vi "Simple UDP - Receiver_.vi"() -> ()   [LabVIEW 2020]
doc: "UDP协议与TCP的区别在于UDP不包括发送数据包信息的错误检查，因此无法保证接收端是否已接收所发数据。\n\nUDP可用于“广播”数据至整个网络，只需指定可包括全部的IP地址(255.255.255.255)以便发送信息至整个网络。 由于路由器或其他网络硬件通常拒绝转发超过一定点的数据，在实际应用中广播范围可能存在限制。"
panel:
  out "波形图表 6":waveform(i32)(graph)
  out "输出波形":waveform(i32)
  in  "停止 2":bool
  out "波形图表 5":i32[](graph)
  in  "服务器关闭":string="服务器VI关闭了连接。"
  # "概述：演示使用UDP函数通过UDP连接接收数据。\n操作步骤：\n1.确保已运行Simple UDP - Sender.vi。\n2.运行VI。\n3.单击停止按钮停止VI。"
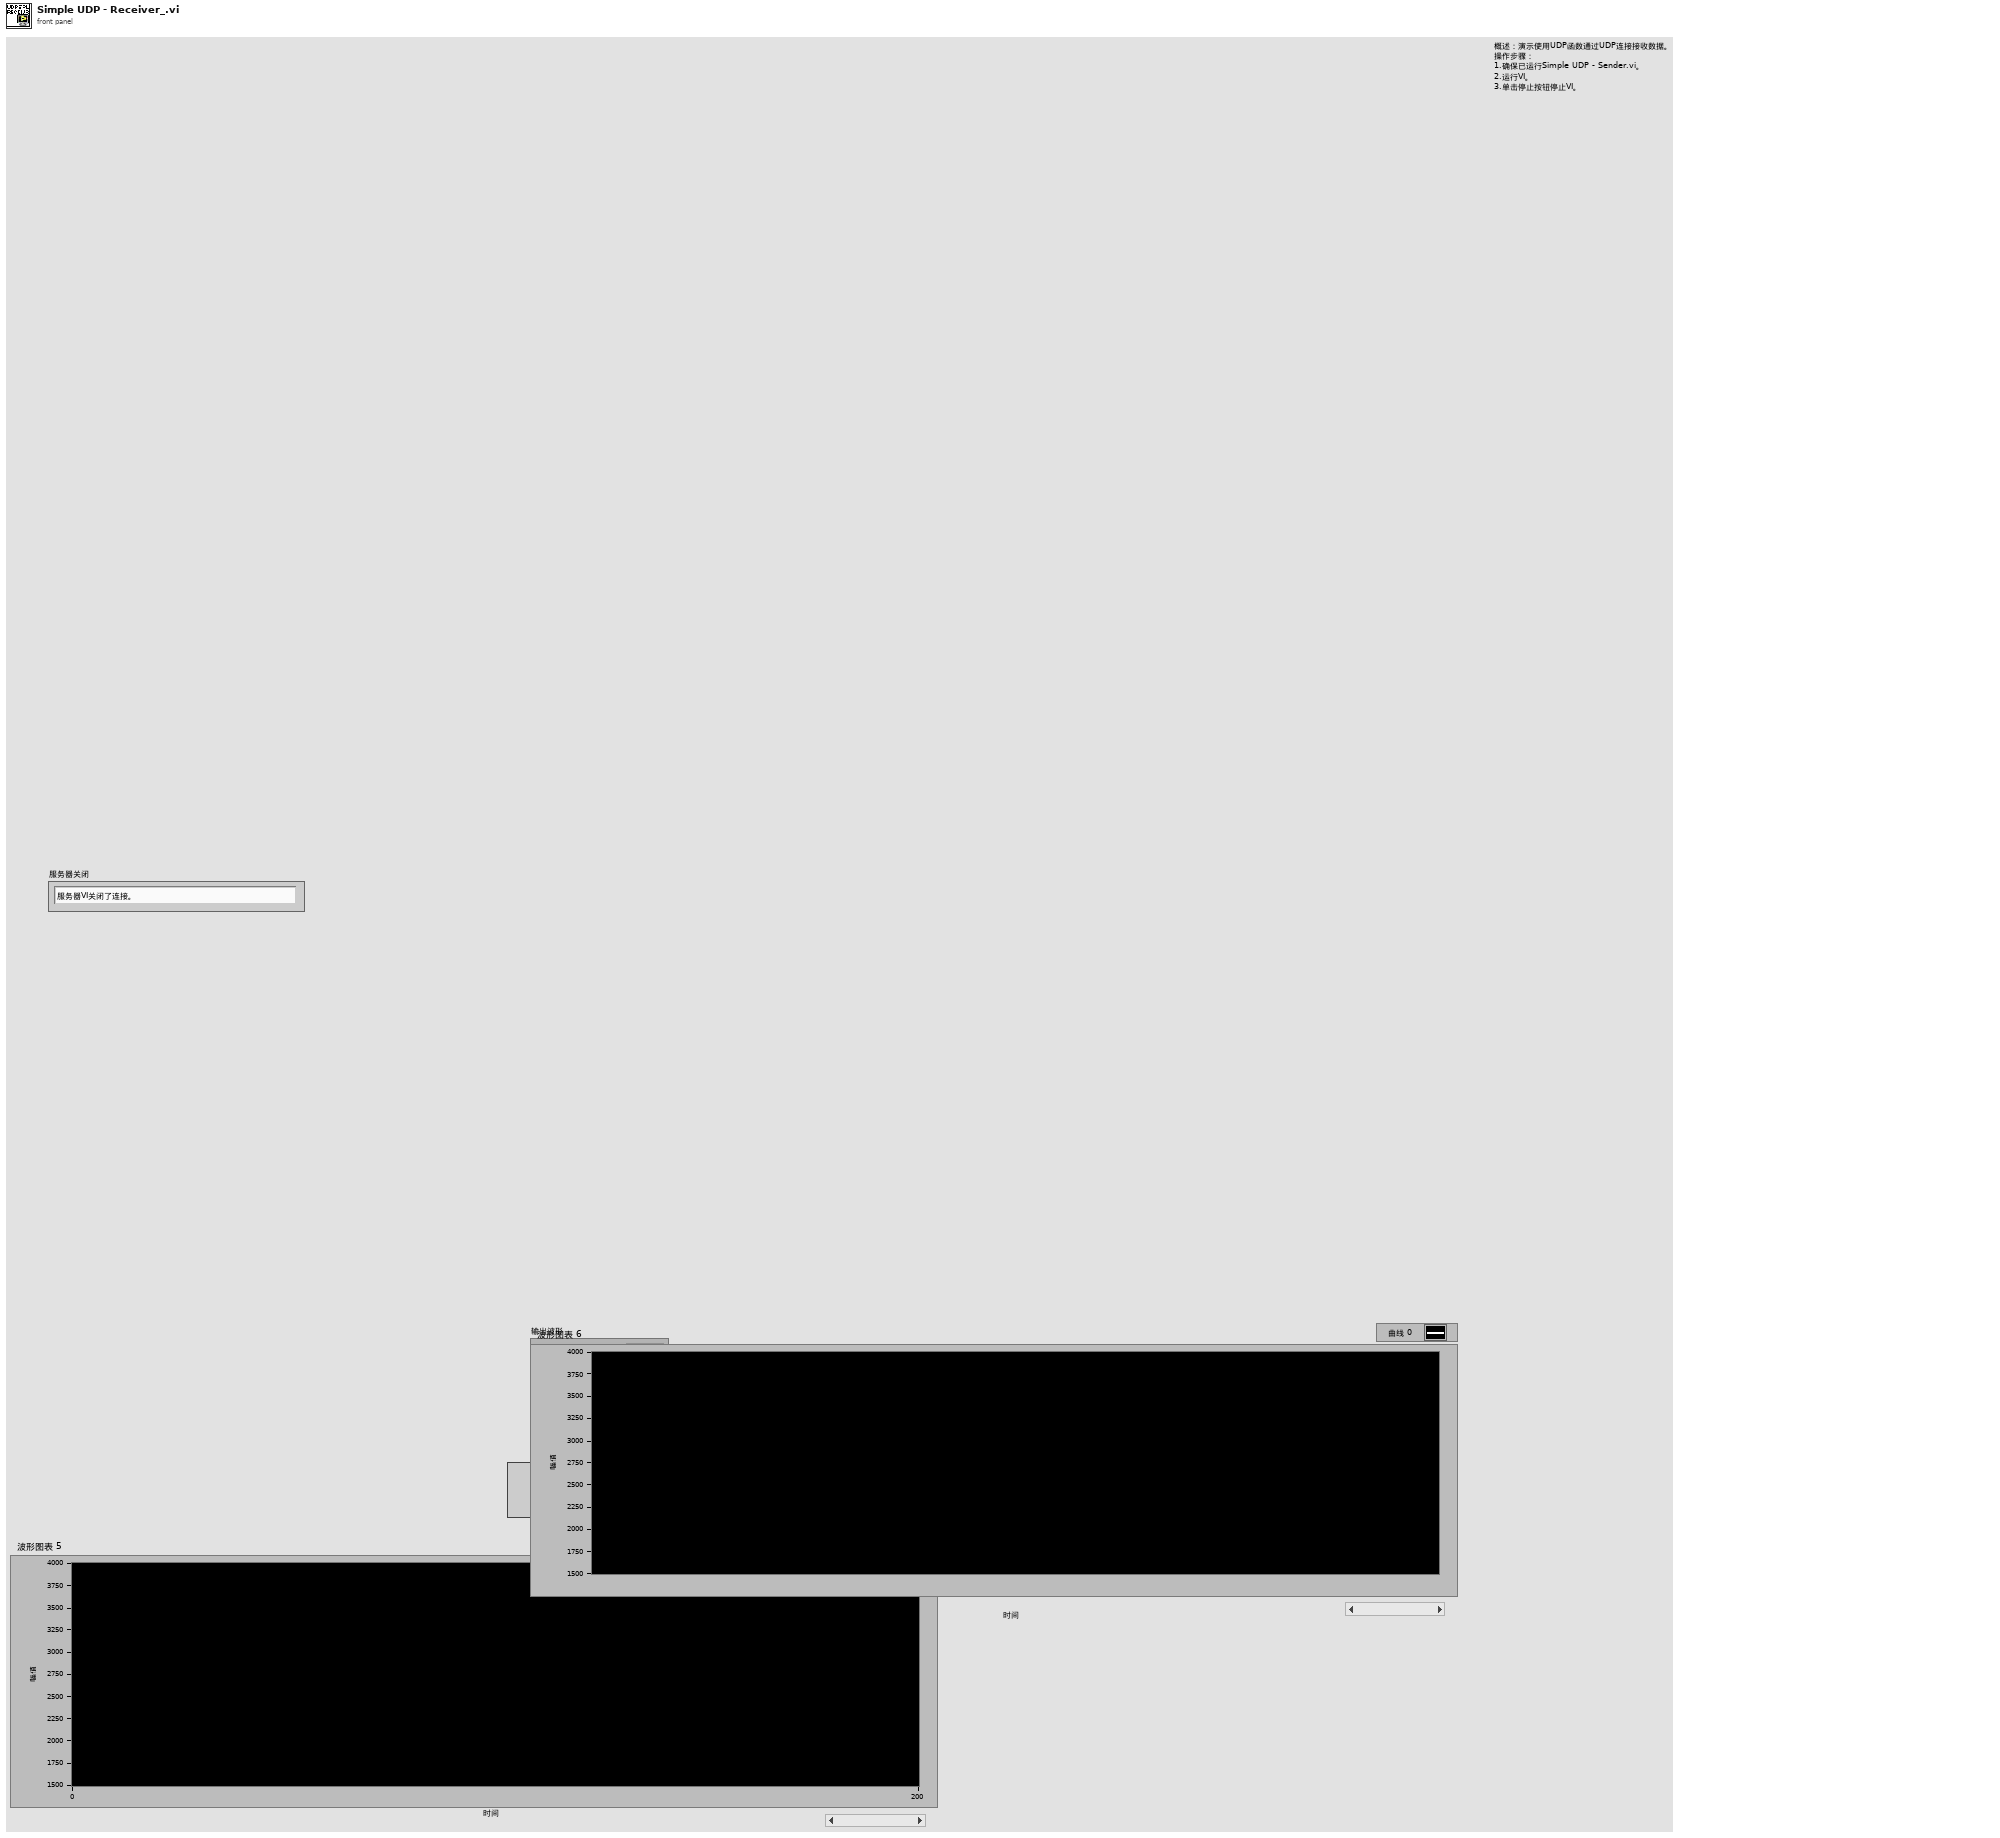
[diagram p1: front panel]
types:
  T1 = enum16{"open", "open or create", "create or replace", "create", "open (read-only)"}
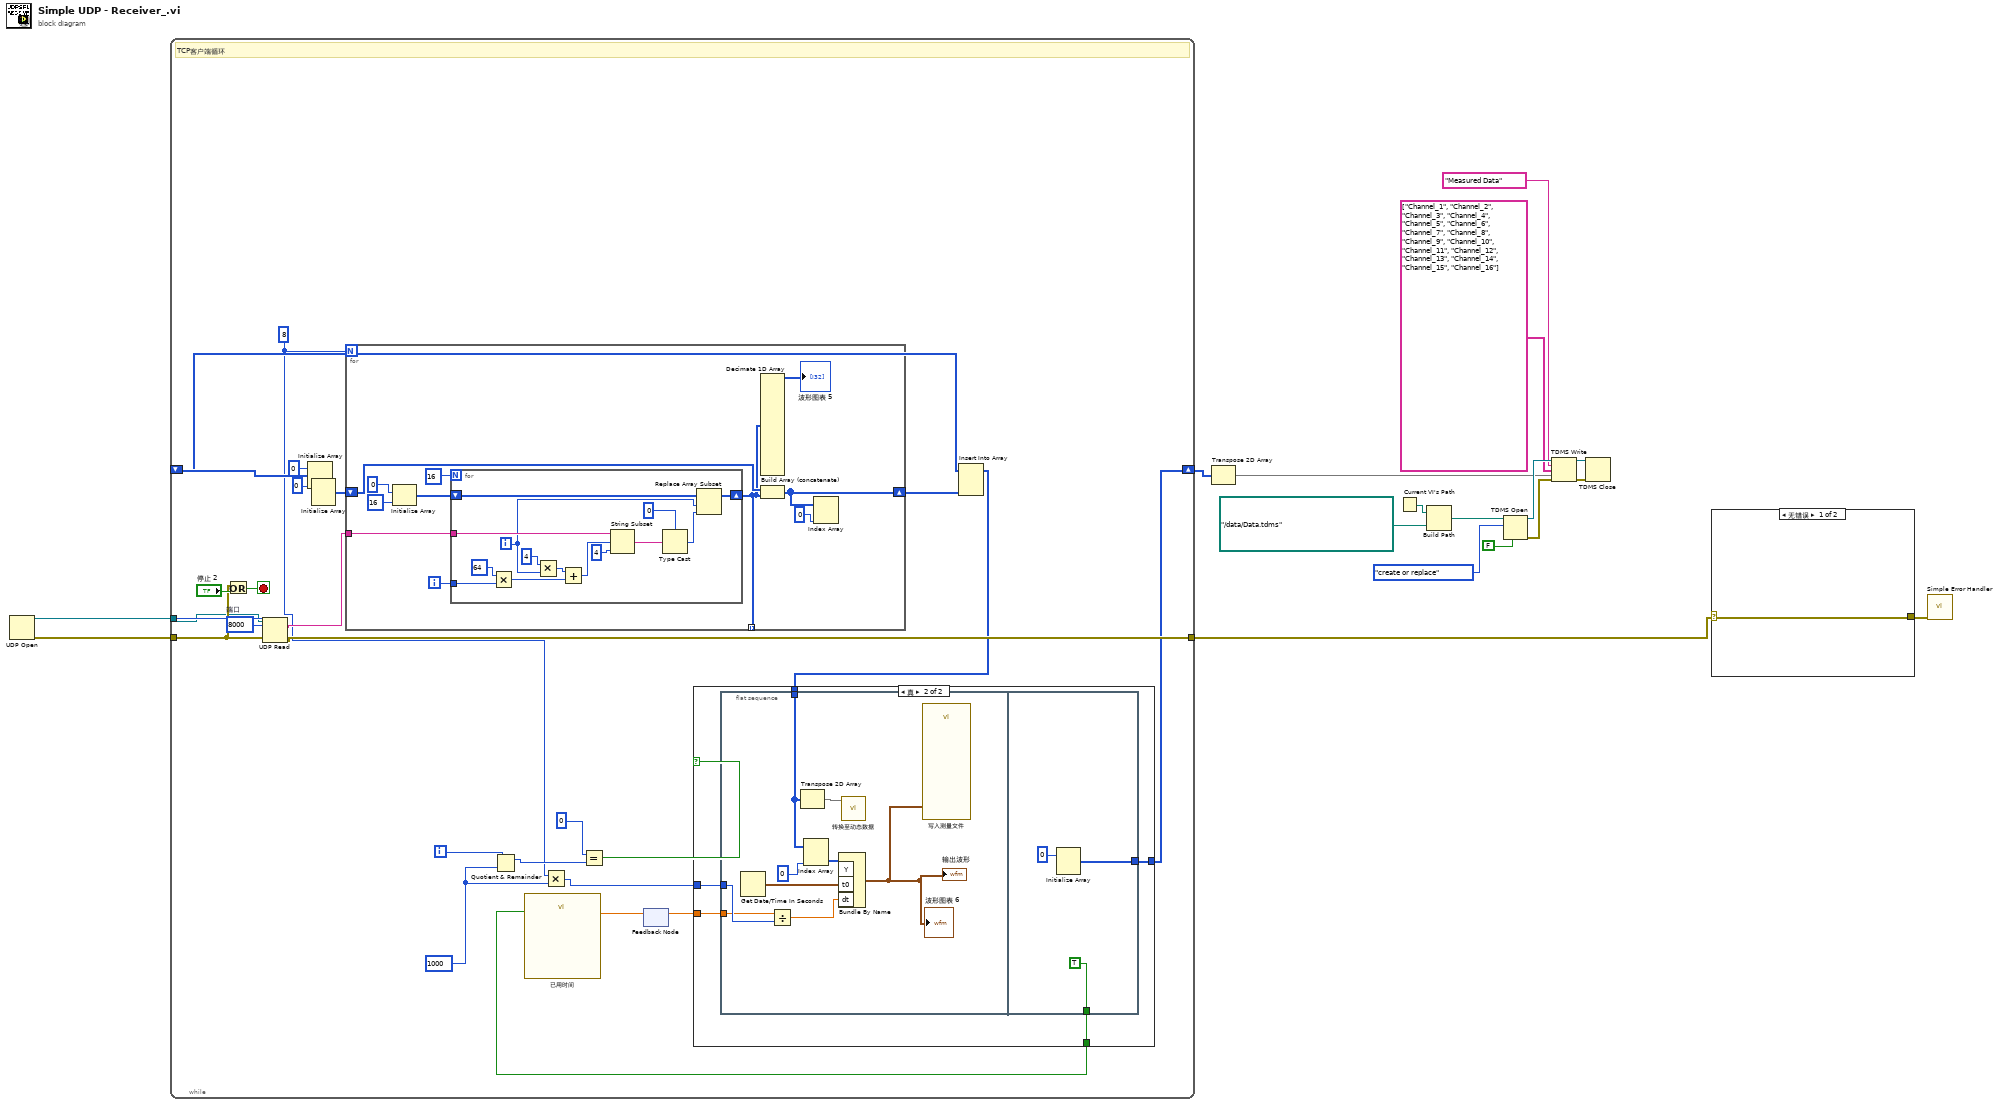
[diagram p0: block diagram]
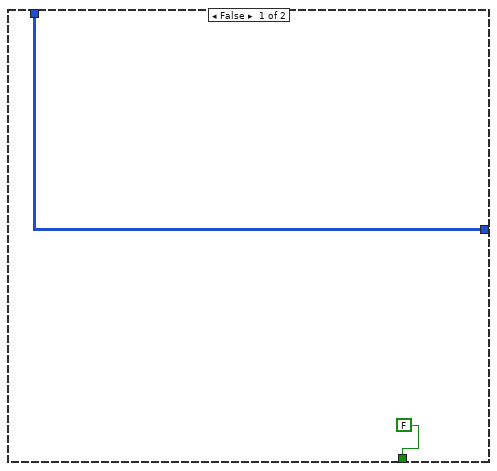
[diagram p2: hidden frame]
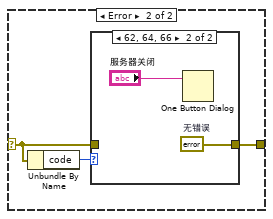
[diagram p3: hidden frame]
diagram:
  w14 = u16 8000  # 端口
  n1 = UDP Open(11:w14) -> (port=w16:refnum<k16>, 0:w15:errorcluster)  [unwired: 4 in, 1 out]
  n2 = Initialize Array(0) -> (w18:i32[][])  [unwired: 2 in]
  n3 = while {
    tunnel: w15 -> [w34]
    tunnel: w16 -> [w33]
    tunnel: [w35] -> w1
    shift-right: [w27] -> w17
    shift-left: w18 -> [w38]
    i -> [w32]
    stop <- w37 stop-if-true
    w23 = 1000
    w22 = u16 8
    # "TCP客户端循环"
    n4 = Or(x=w34, y="停止 2") -> (x .or. y?=w37:bool)
    n5 = UDP Read(connection ID=w33, 8:w34) -> (data out=w36:string, error out=w35:errorcluster)  [unwired: 1 in, 4 out]
    n6 = Initialize Array(0) -> (w40:i32[][])  [unwired: 2 in]
    n7 = for {
      N: w22 -> [_]
      tunnel: w36 -> [w72]
      shift-right: [w65] -> w39
      shift-left: w40 -> [w66]
      tunnel: [w62] -> _ mode=indexing
      i -> [w67]
      n8 = Initialize Array(0, 16) -> (w68:i32[])
      n9 = for {
        N: i8 16 -> [_]
        tunnel: w72 -> [w84]
        tunnel: w67 -> [w80]
        shift-right: [w73] -> w62
        shift-left: w68 -> [w74]
        i -> [w75]
        n10 = Multiply(x=i8 64, y=w80) -> (x*y=w79:i32)
        n11 = Multiply(x=i8 4, y=w75) -> (x*y=w77:i32)
        n12 = Add(x=w77, y=w79) -> (x+y=w78:i32)
        n13 = String Subset(string=w84, offset (0)=w78, length (rest)=i8 4) -> (substring=w86:string)
        n14 = Type Cast(type=0, x=w86) -> (*(type *) &x=w76:i32)
        n15 = Replace Array Subset(array=w74, new element=w76, index=w75) -> (w73:i32[])
      }
      n16 = Decimate 1D Array(w62) -> (→"波形图表 5":i32[])  [unwired: 15 out]
      n17 = Build Array (concatenate)(w66, w62) -> (w65:i32[][])
      n18 = Index Array(array=w65, index (col)=0) -> ()  [unwired: 1 in, 1 out]
    }
    n19 = Quotient & Remainder(x=w32, y=w23) -> (x-y*floor(x/y)=w29:i32)  [unwired: 1 out]
    n20 = Multiply(x=w22, y=w23) -> (x*y=w21:i32)
    n21 = Equal?(x=0, y=w29) -> (x = y?=w30:bool)
    n22 = feedback #1() -> (w24:dbl)  [unwired: 1 in]
    n23 = Insert Into Array(array=w38, new element=w39) -> (w28:i32[][])  [unwired: 2 in]
    n24 = case shown="真" w30 {
      tunnel: w28 -> [w44 w49]
      tunnel: [w44 w48] -> w27
      tunnel: [FALSE w47] -> w26
      tunnel: w21 -> [_ w46]
      tunnel: w24 -> [_ w45]
      frame False {
      }
      frame True {
        n25 = flat-sequence {
          tunnel: w49 -> [w57]
          tunnel: w46 -> [w52]
          tunnel: w45 -> [w50]
          tunnel: [w60] -> w48
          tunnel: [TRUE] -> w47
          frame #0 {
            n26 = Get Date/Time In Seconds() -> (seconds since 1Jan1904=w53:timestamp)
            n27 = Divide(x=w50, y=w52) -> (x/y=w51:dbl)
            n28 = Transpose 2D Array(2D array=w57) -> (transposed array=w58:i32[][])
            n29 = Index Array(array=w57, index (col)=0) -> (element=w56:i32[])  [unwired: 1 in]
            n30 = Bundle By Name ("创建波形")("Y"=w56, "t0"=w53, "dt"=w51) -> (w54:waveform(i32))  [unwired: 1 in]
            "输出波形" <- w54
            "波形图表 6" <- w54
            n31 = call "转换至动态数据"("2D Array"=w58) -> ()  [unwired: 3 in, 1 out]
            n32 = call "写入测量文件"("Signals"=w54) -> ()  [unwired: 16 in, 3 out]
          }
          frame #1 {
            n33 = Initialize Array(0) -> (w60:i32[][])  [unwired: 2 in]
          }
        }
      }
    }
    n34 = call "已用时间"("Reset"=w26) -> ("Elapsed Time (s)"=w25:dbl)  [unwired: 11 in, 7 out]
    n35 = feedback-in #1(w25) -> ()
  }
  n36 = Transpose 2D Array(2D array=w17) -> (transposed array=w3:i32[][])
  n37 = Current VI's Path() -> (path=w2:path)
  n38 = Build Path(base path=w2, name or relative path=path "../data/Data.tdms" ("file path")) -> (appended path=w9:path)
  n39 = TDMS Open(6:FALSE ("disable buffering (T)"), 10:T1."create or replace" ("operation"), 11:w9) -> (0:w13:errorcluster, 3:w10:refnum<k34>)  [unwired: 4 in]
  n40 = TDMS Write(0:w10, 5:"Measured Data" ("group name"), 7:string[] ["Channel_1", "Channel_2", "Channel_3", "Channel_4", "Channel_5", "Channel_6", "Channel_7", "Channel_8", "Channel_9", "Channel_10", "Channel_11", "Channel_12", "Channel_13", "Channel_14", "Channel_15", "Channel_16"] ("channel names"), 9:w3, 11:w13) -> (4:w11:refnum<k34>, 15:w12:errorcluster)  [unwired: 1 in, 2 out]
  n41 = TDMS Close(8:w12, 11:w11) -> ()  [unwired: 2 out]
  n42 = case shown="无错误" w1 {
    selector: w1 -> [w87 w89]
    tunnel: [w87 w88] -> w20
    frame No Error {
    }
    frame Error {
      n43 = Unbundle By Name(w89) -> ("code"=w90:i32)
      n44 = case shown="62, 64, 66" w90 {
        tunnel: w89 -> [w91 _]
        tunnel: [w91 w93] -> w88
        frame Default {
        }
        frame 62, 64, 66 {
          w93 = errorcluster {"status"=FALSE, "code"=0, "source"=""}  # 无错误
          n45 = One Button Dialog(message="服务器关闭") -> ()  [unwired: 1 in, 1 out]
        }
      }
    }
  }
  n46 = call <vilib>:"Simple Error Handler.vi"("error in (no error)"=w20) -> ()  [unwired: 4 in, 5 out]
